vi "Probe_DATA_COM.vi"() -> ()   [LabVIEW 2019]
uses:
  <vilib>/Instr/_visa.llb/VISA Configure Serial Port (Instr).vi
panel:
  in  "stop":bool
  out "read buffer":string
  in  "VISA resource name":refnum<visa-resource-name>
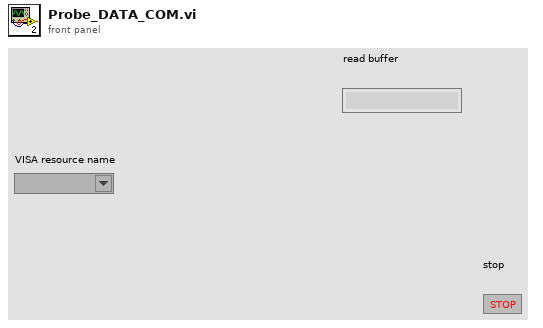
[diagram p1: front panel]
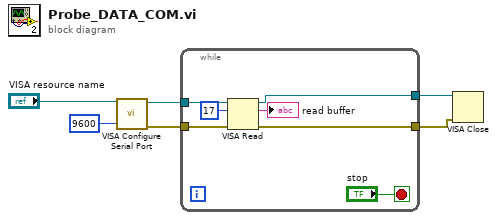
[diagram p0: block diagram]
diagram:
  n1 = call-poly "VISA Configure Serial Port"("VISA resource name"="VISA resource name", "baud rate (9600)"=u32 9600) -> ("VISA resource name out"=w6:refnum<visa-resource-name>, "error out"=w5:errorcluster)  [unwired: 12 in]
  n2 = while {
    tunnel: w6 -> [w13]
    tunnel: w5 -> [w12]
    tunnel: [w9] -> w2
    tunnel: [w8] -> w1
    stop <- "stop" stop-if-true
    n3 = VISA Read(VISA resource name=w13, byte count=u32 17, error in (no error)=w12) -> (VISA resource name out=w8:refnum<visa-resource-name>, read buffer=→"read buffer":string, error out=w9:errorcluster)  [unwired: 1 out]
  }
  n4 = VISA Close(VISA resource name=w1, error in (no error)=w2) -> ()  [unwired: 1 out]
